vi "Register Metric.vi"(8 "error in (no error)":errorcluster, 9 "New Metric":refnum<data-value>, 11 "Session Handle in":T1) -> (0 "error out":errorcluster, 3 "Session Handle out":T1)   [LabVIEW 2020, in "Registry.lvlib" / "Registry Session.lvclass"]
uses:
  Registry Session.lvclass
  Typedefs/Session Handle.ctl
  metrics/metric/Metric.lvclass
  metrics/metric/Metric.lvclass/Metric.ctl
  Registry Session.lvclass/Registry Session.ctl
  metrics/metric/Read Name.vi
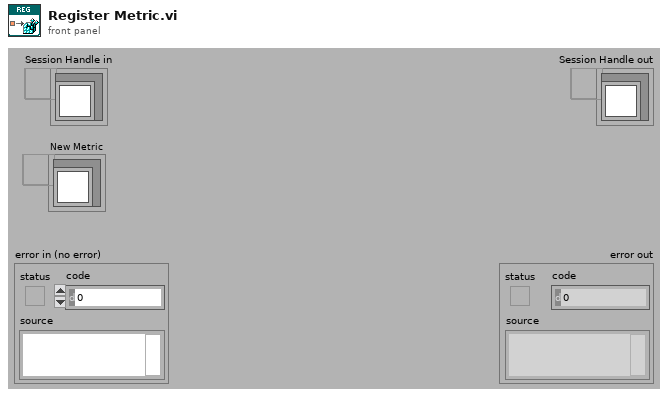
[diagram p1: front panel]
types:
  T1 = typedef "Registry.lvlib/Registry Session.lvclass/Session Handle.ctl" = refnum<data-value>
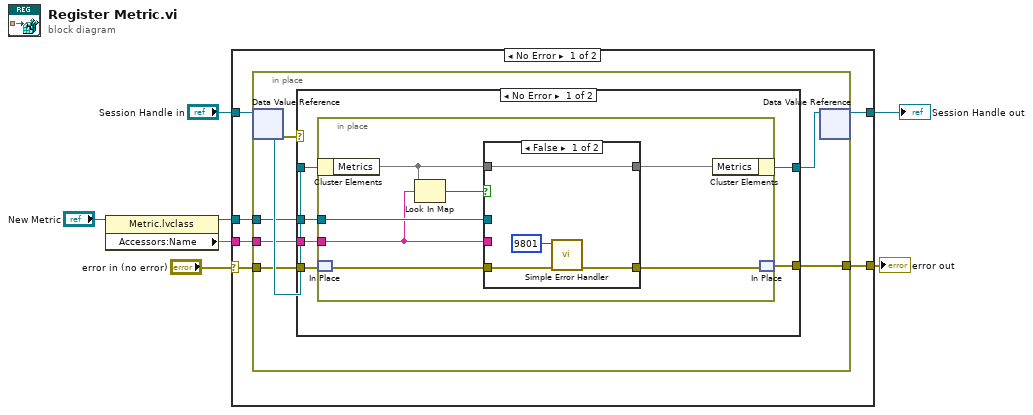
[diagram p0: block diagram]
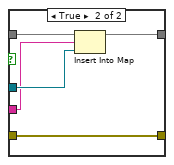
[diagram p2: hidden frame]
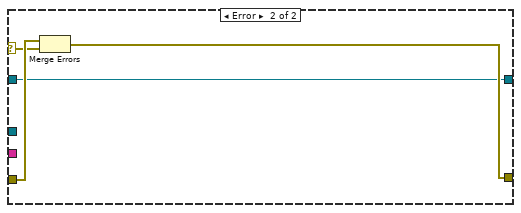
[diagram p3: hidden frame]
diagram:
  n1 = property class="Metric.lvclass"(reference="New Metric") -> (reference out=w1:refnum<data-value>, "Accessors:Name"=w2:string)  [unwired: 1 in, 1 out]
  n2 = case shown="No Error" "error in (no error)" {
    selector: "error in (no error)" -> [w11 w47]
    tunnel: "Session Handle in" -> [w13 w48]
    tunnel: [w12 w48] -> w6
    tunnel: [w10 w47] -> w5
    tunnel: w1 -> [w9 _]
    tunnel: w2 -> [w8 _]
    frame No Error {
      n3 = in-place {
        in-place-border: w11 -> [w16]
        in-place-border: [w19] -> w10
        in-place-border: w9 -> [w15]
        in-place-border: w8 -> [w14]
        n4 = in-place-dvr #1(w13) -> (w20:refnum<class "Registry Session.lvclass">, w17:errorcluster)
        n5 = case shown="No Error" w17 {
          selector: w17 -> [_ w45]
          tunnel: w20 -> [w25 w43]
          tunnel: [w21 w44] -> w19
          tunnel: [w24 w43] -> w18
          tunnel: w16 -> [w22 w46]
          tunnel: w15 -> [w26 _]
          tunnel: w14 -> [w23 _]
          frame No Error {
            n6 = in-place {
              in-place-border: w26 -> [w33]
              in-place-border: w23 -> [w32]
              n7 = in-place-cluster #2(w25) -> ("Metrics"=w31:map{string, refnum<data-value>})
              n8 = in-place-match #3(w22) -> (w27:errorcluster)
              n9 = Look In Map(map=w31, key=w32) -> (key not found?=w29:bool)  [unwired: 1 in, 1 out]
              n10 = case shown="False" w29 {
                tunnel: w33 -> [_ w42]
                tunnel: w32 -> [_ w41]
                tunnel: w31 -> [w37 w40]
                tunnel: [w37 w39] -> w30
                tunnel: [w34 w38] -> w28
                tunnel: w27 -> [w36 w38]
                frame False {
                  n11 = call <vilib>:"Simple Error Handler.vi"("error code (no error:0)"=9801, "error in (no error)"=w36) -> ("error out"=w34:errorcluster)  [unwired: 3 in, 4 out]
                }
                frame True {
                  n12 = Insert Into Map(map in=w40, key=w41, value=w42) -> (map out=w39:map{string, refnum<data-value>})  [unwired: 2 out]
                }
              }
              n13 = in-place-cluster #2("Metrics"=w30) -> (w24:refnum<class "Registry Session.lvclass">)
              n14 = in-place-match #3(w28) -> (w21:errorcluster)
            }
          }
          frame Error {
            n15 = Merge Errors(w46, w45) -> (w44:errorcluster)
          }
        }
        n16 = in-place-dvr #1(w18) -> (w12:T1)  [unwired: 1 out]
      }
    }
    frame Error {
    }
  }
  "Session Handle out" <- w6
  "error out" <- w5
